vi "Refill.vi"(8 "Error In":errorcluster, 10 "MedicalDroid In":refnum<class "MedicalDroid.lvclass">, 11 "BactaTank in":refnum<class "BactaTank.lvclass">) -> (0 "Error Out":errorcluster, 2 "MedicalDroid Out":refnum<class "MedicalDroid.lvclass">, 3 "BactaTank out":refnum<class "BactaTank.lvclass">)   [LabVIEW 2021, in "BactaTank.lvclass"]
uses:
  BactaTank.lvclass
  MedicalDroid/MedicalDroid.lvclass
  BactaTank.lvclass/BactaTank.ctl
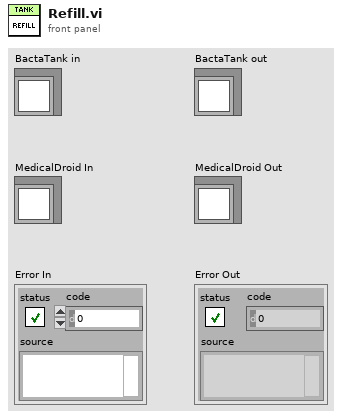
[diagram p1: front panel]
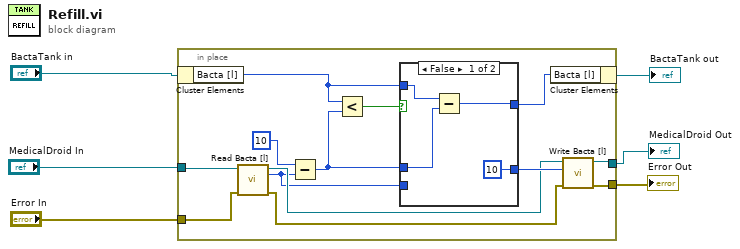
[diagram p0: block diagram]
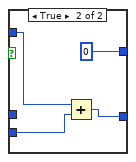
[diagram p2: hidden frame]
diagram:
  n1 = in-place {
    in-place-border: "Error In" -> [w17]
    in-place-border: "MedicalDroid In" -> [w19]
    in-place-border: [w10] -> w2
    in-place-border: [w9] -> w3
    n2 = in-place-cluster #1("BactaTank in") -> ("Bacta [l]"=w15:u8)
    n3 = call "Read Bacta [l].vi"("error in (no error)"=w17, "MedicalDroid in"=w19) -> ("error out"=w11:errorcluster, "Bacta [l]"=w7:u8, "MedicalDroid out"=w12:refnum<class "MedicalDroid.lvclass">)  [unwired: 7 in]
    n4 = Subtract(x=u8 10, y=w7) -> (x-y=w14:u8)
    n5 = Less?(x=w15, y=w14) -> (x < y?=w16:bool)
    n6 = case shown="False" w16 {
      tunnel: w15 -> [w22 w27]
      tunnel: w14 -> [w21 _]
      tunnel: [u8 10 w26] -> w13
      tunnel: [w20 u8 0] -> w8
      tunnel: w7 -> [_ w24]
      frame False {
        n7 = Subtract(x=w22, y=w21) -> (x-y=w20:u8)
      }
      frame True {
        n8 = Add(x=w27, y=w24) -> (x+y=w26:u8)
      }
    }
    n9 = in-place-cluster #1("Bacta [l]"=w8) -> (→"BactaTank out":refnum<class "BactaTank.lvclass">)
    n10 = call "Write Bacta [l].vi"("error in (no error)"=w11, "Bacta [l]"=w13, "MedicalDroid in"=w12) -> ("error out"=w9:errorcluster, "MedicalDroid out"=w10:refnum<class "MedicalDroid.lvclass">)  [unwired: 7 in]
  }
  "Error Out" <- w3
  "MedicalDroid Out" <- w2
